vi "Init_ImagesV2.vi"() -> (3 "Images":T1)   [LabVIEW 2011]
uses:
  Image ClusterV2.ctl
  <vilib>/vision/Image Controls.llb/IMAQ Image.ctl
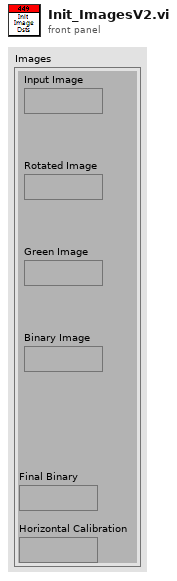
[diagram p1: front panel]
types:
  T1 = typedef "Image ClusterV2.ctl" = cluster{"Input Image":T2, "Rotated Image":T2, "Green Image":T2, "Binary Image":T2, "Final Binary":T2, "Horizontal Calibration":T2}
  T2 = typedef "IMAQ Image.ctl" = refnum<image>
  T3 = typedef "Image Type" = u32
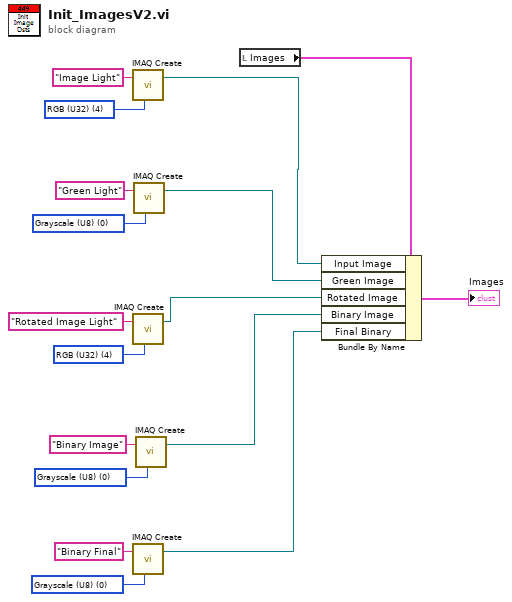
[diagram p0: block diagram]
diagram:
  w3 = T3 0 items=["Grayscale (U8)", "Grayscale (I16)", "Grayscale (SGL)", "Complex (CSG)", "RGB (U32)", "HSL (U32)", "RGB (U64)", "Grayscale (U16)"] ("Image Type")
  w4 = T3 4 items=["Grayscale (U8)", "Grayscale (I16)", "Grayscale (SGL)", "Complex (CSG)", "RGB (U32)", "HSL (U32)", "RGB (U64)", "Grayscale (U16)"] ("Image Type")
  w7 = T3 0 items=["Grayscale (U8)", "Grayscale (I16)", "Grayscale (SGL)", "Complex (CSG)", "RGB (U32)", "HSL (U32)", "RGB (U64)", "Grayscale (U16)"] ("Image Type")
  w14 = T3 0 items=["Grayscale (U8)", "Grayscale (I16)", "Grayscale (SGL)", "Complex (CSG)", "RGB (U32)", "HSL (U32)", "RGB (U64)", "Grayscale (U16)"] ("Image Type")
  w16 = T3 4 items=["Grayscale (U8)", "Grayscale (I16)", "Grayscale (SGL)", "Complex (CSG)", "RGB (U32)", "HSL (U32)", "RGB (U64)", "Grayscale (U16)"] ("Image Type")
  n1 = call "IMAQ Create"("Image Name"="Image Light", "Image Type"=w4) -> ("New Image"=w10:T2)  [unwired: 3 in, 1 out]
  n2 = call "IMAQ Create"("Image Name"="Rotated Image Light", "Image Type"=w16) -> ("New Image"=w8:T2)  [unwired: 3 in, 1 out]
  n3 = call "IMAQ Create"("Image Name"="Binary Final", "Image Type"=w3) -> ("New Image"=w1:T2)  [unwired: 3 in, 1 out]
  n4 = call "IMAQ Create"("Image Name"="Green Light", "Image Type"=w14) -> ("New Image"=w9:T2)  [unwired: 3 in, 1 out]
  n5 = call "IMAQ Create"("Image Name"="Binary Image", "Image Type"=w7) -> ("New Image"=w5:T2)  [unwired: 3 in, 1 out]
  n6 = local read "Images"() -> (w12:T1)
  n7 = Bundle By Name(cluster=w12, "Input Image"=w10, "Green Image"=w9, "Rotated Image"=w8, "Binary Image"=w5, "Final Binary"=w1) -> (→"Images":T1)
